vi "Error Main.vi"(8 "error in (no error)":errorcluster) -> (0 "error out":errorcluster)   [LabVIEW 2020, in "Error handler.lvlib"]
doc: "This is the Main VI for the Error handler Module."
uses:
  Error handler.lvlib
  Private Controls/FG Actions.ctl
  Private Controls/Message enum.ctl
  Private Controls/Message Cluster.ctl
  Private Controls/Module Data.ctl
  ATM Controller/ATM_Controller.lvlib
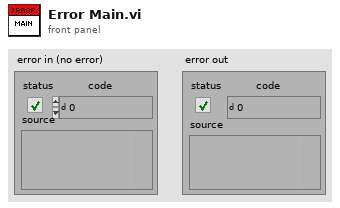
[diagram p1: front panel]
types:
  T1 = typedef "Error handler.lvlib/Module Data.ctl" = cluster{"Data":variant}
  T2 = typedef "Error handler.lvlib/FG Actions.ctl" = enum16{"Get", "Set", "Clear"}
  T3 = typedef "Error handler.lvlib/Message Cluster.ctl" = cluster{"Message":T4, "Data":variant}
  T4 = typedef "Error handler.lvlib/Message enum.ctl" = enum16{"Initialize", "State", "Error", "Exit", "Log", "Process_Sensor_Error", "Display_Console_Error", "User_Console_Error"}
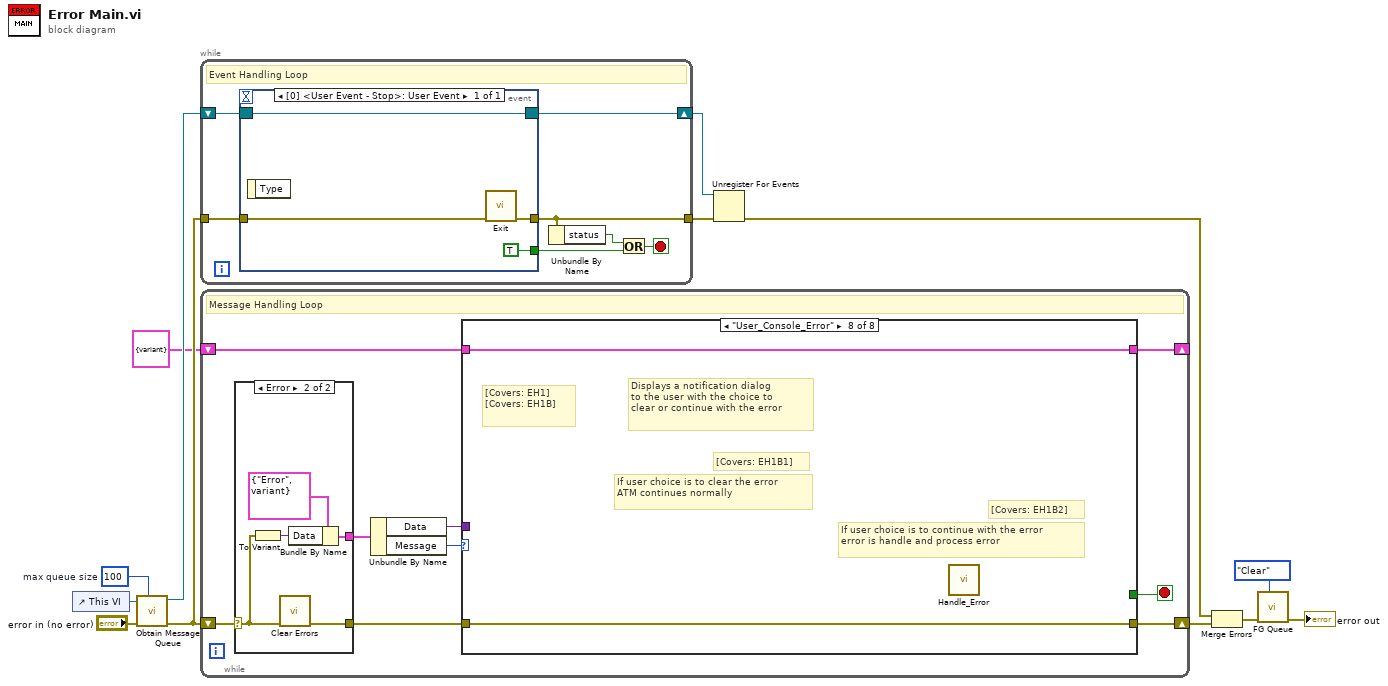
[diagram p0: block diagram]
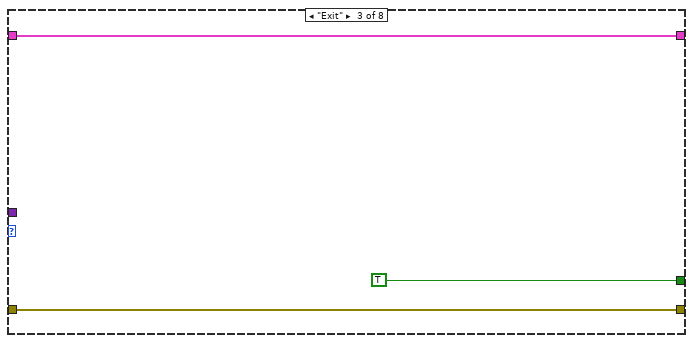
[diagram p4: hidden frame]
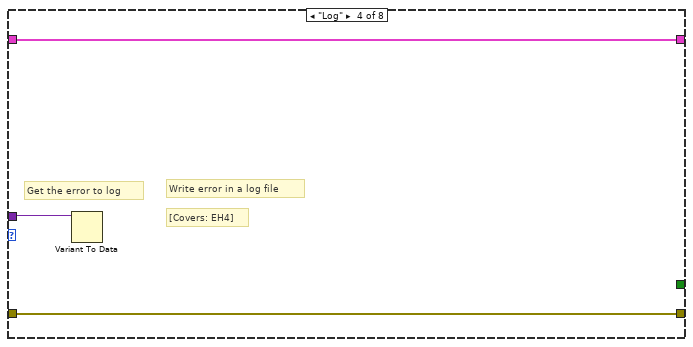
[diagram p5: hidden frame]
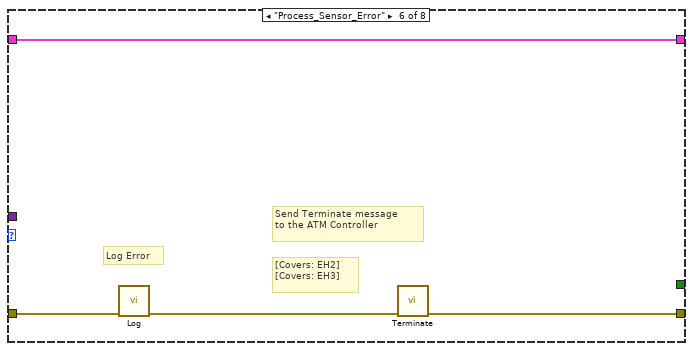
[diagram p7: hidden frame]
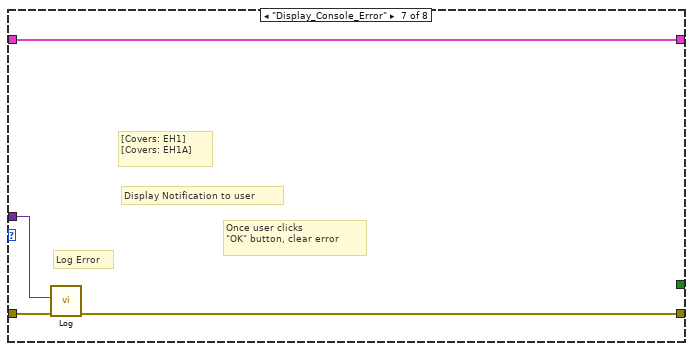
[diagram p8: hidden frame]
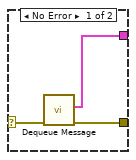
[diagram p9: hidden frame]
diagram:
  w7 = 100  # max queue size
  n1 = control-ref of="This VI"() -> (w8:refnum<vi>)
  n2 = call "Obtain Message Queue.vi"("max queue size (-1, unlimited)"=w7, "error in (no error)"="error in (no error)", "VI Reference"=w8) -> ("error out"=w3:errorcluster, "Event Registration Refnum"=w10:refnum<event-registration>)  [unwired: 7 in]
  n3 = while {
    shift-right: [w19] -> w11
    shift-left: w10 -> [w20]
    tunnel: w3 -> [w17]
    tunnel: [w15] -> w2
    stop <- w16 stop-if-true
    # "Event Handling Loop"
    n4 = event shown="[0] <User Event - Stop>: User Event" {
      selector: w20 -> [w21]
      dyn-events: [w21] -> w19
      timeout: _ -> [_]
      tunnel: [TRUE ("Discard?")] -> w18
      tunnel: w17 -> [w23]
      tunnel: [w22] -> w15
      event User Event {
        n5 = event-data() -> ()  [unwired: 1 in, 1 out]
        n6 = call "Exit.vi"("error in (no error)"=w23) -> ("error out"=w22:errorcluster)  [unwired: 10 in]
      }
    }
    n7 = Unbundle By Name(w15) -> ("status"=w14:bool)
    n8 = Or(x=w14, y=w18) -> (x .or. y?=w16:bool)
  }
  n9 = while {
    shift-right: [w28] -> w13
    shift-left: w3 -> [w33]
    shift-right: [w25] -> _
    shift-left: T1 {"Data"=variant} ("Message Cluster") -> [w26]
    stop <- w27 stop-if-true
    # "Message Handling Loop"
    n10 = case shown="Error" w33 {
      selector: w33 -> [w56 w62]
      tunnel: [w57 w63] -> w29
      tunnel: [w58 w59] -> w32
      frame No Error {
        n11 = call "Dequeue Message.vi"("error in (no error)"=w56) -> ("error out"=w57:errorcluster, "Element"=w58:T3)  [unwired: 9 in]
      }
      frame Error {
        n12 = To Variant(anything=w62) -> (Variant=w60:variant)
        n13 = call <vilib>:"Clear Errors.vi"("error in (no error)"=w62) -> ("error out"=w63:errorcluster)  [unwired: 5 in, 1 out]
        n14 = Bundle By Name(cluster=T3 {"Message"=enum."Error", "Data"=variant} ("Message Cluster"), "Data"=w60) -> (w59:T3)
      }
    }
    n15 = Unbundle By Name(w32) -> ("Data"=w30:variant, "Message"=w31:T4)
    n16 = case shown="\"User_Console_Error\"" w31 {
      tunnel: w30 -> [_ _ _ w41 _ _ w52 _]
      tunnel: w29 -> [w35 w37 w40 w43 w45 w47 w51 w55]
      tunnel: [w35 w37 w40 w43 w45 w48 w50 w55] -> w28
      tunnel: [_ _ TRUE _ _ _ _ _] -> w27
      tunnel: w26 -> [w34 w36 w38 w42 w44 w49 w53 w54]
      tunnel: [w34 w36 w38 w42 w44 w49 w53 w54] -> w25
      frame "Initialize", Default {
        # "[Covers: EH4]"
        # "Put File Reference\nin the Module data"
        # "Create Error Log File\nIncluding Error Description\nError Level\nTime and date"
      }
      frame "Error" {
      }
      frame "Exit" {
      }
      frame "Log" {
        # "Write error in a log file"
        # "[Covers: EH4]"
        # "Get the error to log"
        n17 = Variant To Data(Variant=w41) -> ()  [unwired: 2 in, 2 out]
      }
      frame "State" {
      }
      frame "Process_Sensor_Error" {
        # "Log Error"
        # "[Covers: EH2] \n[Covers: EH3]"
        # "Send Terminate message\nto the ATM Controller"
        n18 = call "Log.vi"("error in (no error)"=w47) -> ("error out"=w46:errorcluster)  [unwired: 10 in]
        n19 = call "Terminate.vi"("error in (no error)"=w46) -> ("error out"=w48:errorcluster)  [unwired: 10 in]
      }
      frame "Display_Console_Error" {
        # "[Covers: EH1] \n[Covers: EH1A]"
        # "Log Error"
        # "Once user clicks\n\"OK\" button, clear error"
        # "Display Notification to user"
        n20 = call "Log.vi"("error in (no error)"=w51, "Variant"=w52) -> ("error out"=w50:errorcluster)  [unwired: 9 in]
      }
      frame "User_Console_Error" {
        # "[Covers: EH1B1]"
        # "[Covers: EH1B2]"
        # "If user choice is to continue with the error\nerror is handle and process error"
        # "If user choice is to clear the error\nATM continues normally"
        # "Displays a notification dialog\nto the user with the choice to\nclear or continue with the error"
        # "[Covers: EH1]  \n[Covers: EH1B]"
        n21 = call "Handle_Error.vi"() -> ()  [unwired: 11 in, 1 out]
      }
    }
  }
  n22 = Unregister For Events(event registration refnum=w11, error in=w2) -> (error out=w12:errorcluster)
  n23 = Merge Errors(w12, w13) -> (w5:errorcluster)
  n24 = call "FG Queue.vi"("FG Actions"=FG_Actions."Clear", "error in (no error)"=w5) -> ("error out"=→"error out":errorcluster)  [unwired: 8 in, 1 out]
